vi "Role Playing Simple.vi"(0 "channel":T5, 1 "AI Parameters":T1={"GotoKick"={"Dist do cone a frente"=150.0, "attacker farback"=1500.0, "Perto"=300.0, "min dist to kick"=150.0, "kick eps"=0.0, "Time to transition"=0.05}, "Attacker"={"CC chute"=0.09, "CC passe"=0.045, "Kick Force"=100.0, "D ball-robot Kick"=200.0, "D ball-robot Pass"=0.3}, "Defender"={"D max"=1700.0, "Vel p/ robô av"=1000.0, "Kick Force"=100.0, "D atk-def"=0.0, "D farback"=0.0}, "Timeout"={"Field/v in x"=6.0, "Dist Robots"=300, "Dist up in y"=300}, "Pose Striker"={"dist"=200.0, "Numeric"=-4.0, "dist 2"=200.0}, "Dist Stop"=300.0, "Distance when ball out"=200, "D central gap "=150.0, "T pass"=0.0, "Force ++"=0.0, "range kick"=0.0, "Chute alto"=TRUE, "Marcador novo"=TRUE} {"D central gap" format="%#_13g"; "Dist Stop" format="%#_13g"; "Pose Striker"."Numeric" format="%#_13g"; "Defender"."Kick Force" format="%#_13g"; "Defender"."Vel p/ robô av" format="%#_13g"; "Attacker"."D ball-robot Kick" format="%#_13g"; "Attacker"."Kick Force" format="%#_13g"; "Attacker"."CC passe" format="%#_13g"; "Attacker"."CC chute" format="%#_13g"; "GotoKick"."kick eps" format="%#_13g"; "GotoKick"."min dist to kick" format="%#_13g"; "GotoKick"."Perto" format="%#_13g"; "GotoKick"."attacker farback" format="%#_13g"; "GotoKick"."Dist do cone a frente" format="%#_13g"}, 5 "channel":T4, 9 "test module":T2, 12 "atacando ao contrário?":bool=TRUE) -> (3 "kick \nerror":dbl, 4 "channel":T5, 6 "IA State Output":T6={"our_robots"=[], "enemy_robots"=[], "balls"=[], "geometry"={"line_width"=0, "field_length"=0, "field_width"=0, "boundary_width"=0, "referee_width"=0, "goal_width"=0, "goal_depth"=0, "goal_wall_width"=0, "center_circle_radius"=0, "defense_radius"=0, "defense_stretch"=0, "free_kick_from_defense_dist"=0, "penalty_spot_from_field_line_dist"=0, "penalty_line_from_spot_dist"=0}, "IA Judge"={"stage"="", "command"="", "our_goalie_id"=0.0, "enemy_goalie_id"=0.0, "command enum"=enum."Halt", "Time"=enum."Azul"}, "Received Timestamp"=timestamp(0 s since 1904-01-01), "Events"={"Touch"=FALSE, "Ball out"=FALSE, "id touch"=0.0, "Ball out of \nVision"=FALSE, "Ball inside \nGoalie area"=FALSE, "Robot not responding"=FALSE, "Robots responding status"=[1.0, 1.0, 1.0, 1.0, 1.0, 1.0], "Enemy Ball \nPossession"=FALSE, "Pass State"=FALSE, "id end of pass"=0.0, "Kick"=FALSE, "Id ini Possession"=0.0, "Ball Possesion"=FALSE, "Id Possesion"=0.0}}, 10 "channel to field":T5, 14 "ball":dbl(graph), 15 "Robot":dbl(graph))   [LabVIEW 2017]
uses:
  <extravilib>/ChannelInstances/Lossy Stream-t'AI Input.ctl'/)Channel.ctl
  Core/AI Input.ctl
  Core/AI Robot.ctl
  Intel/Functions Enum.ctl
  Intel/AttackerStates.ctl
  Core/AI Ball.ctl
  Core/Field Size.ctl
  Core/AI Judge.ctl
  Intel/Command Enum.ctl
  Util/Events/Events.ctl
  <extravilib>/ChannelInstances/Lossy Stream-a[.](i32)/)Channel.ctl
  Test/TestModule.ctl
  Util/Select None or Robot.ctl
  Intel/AI Parameters.ctl
  <extravilib>/ChannelInstances/Lossy Stream-a[.](i32)/Read With Abort.vi
  <extravilib>/ChannelInstances/Lossy Stream-t'AI Input.ctl'/Read With Abort.vi
  <extravilib>/ChannelInstances/Lossy Stream-t'AI Input.ctl'/Write With Abort.vi
  <extravilib>/ChannelInstances/Lossy Stream-a[.](i32)/EndpointRead.vi
  <extravilib>/ChannelInstances/Lossy Stream-t'AI Input.ctl'/EndpointRead.vi
  <extravilib>/ChannelInstances/Lossy Stream-t'AI Input.ctl'/Endpoint.vi
  <extravilib>/ChannelInstances/Lossy Stream-t'AI Input.ctl'/)Channel.vi
  <resource>/ChannelSupport/_ChannelSupport/WaitIfNeeded.vi
  <extravilib>/ChannelInstances/Lossy Stream-a[.](i32)/)Channel.vi
  <extravilib>/ChannelInstances/Lossy Stream-t'AI Input.ctl'.lvlib
  <extravilib>/ChannelInstances/Lossy Stream-a[.](i32).lvlib
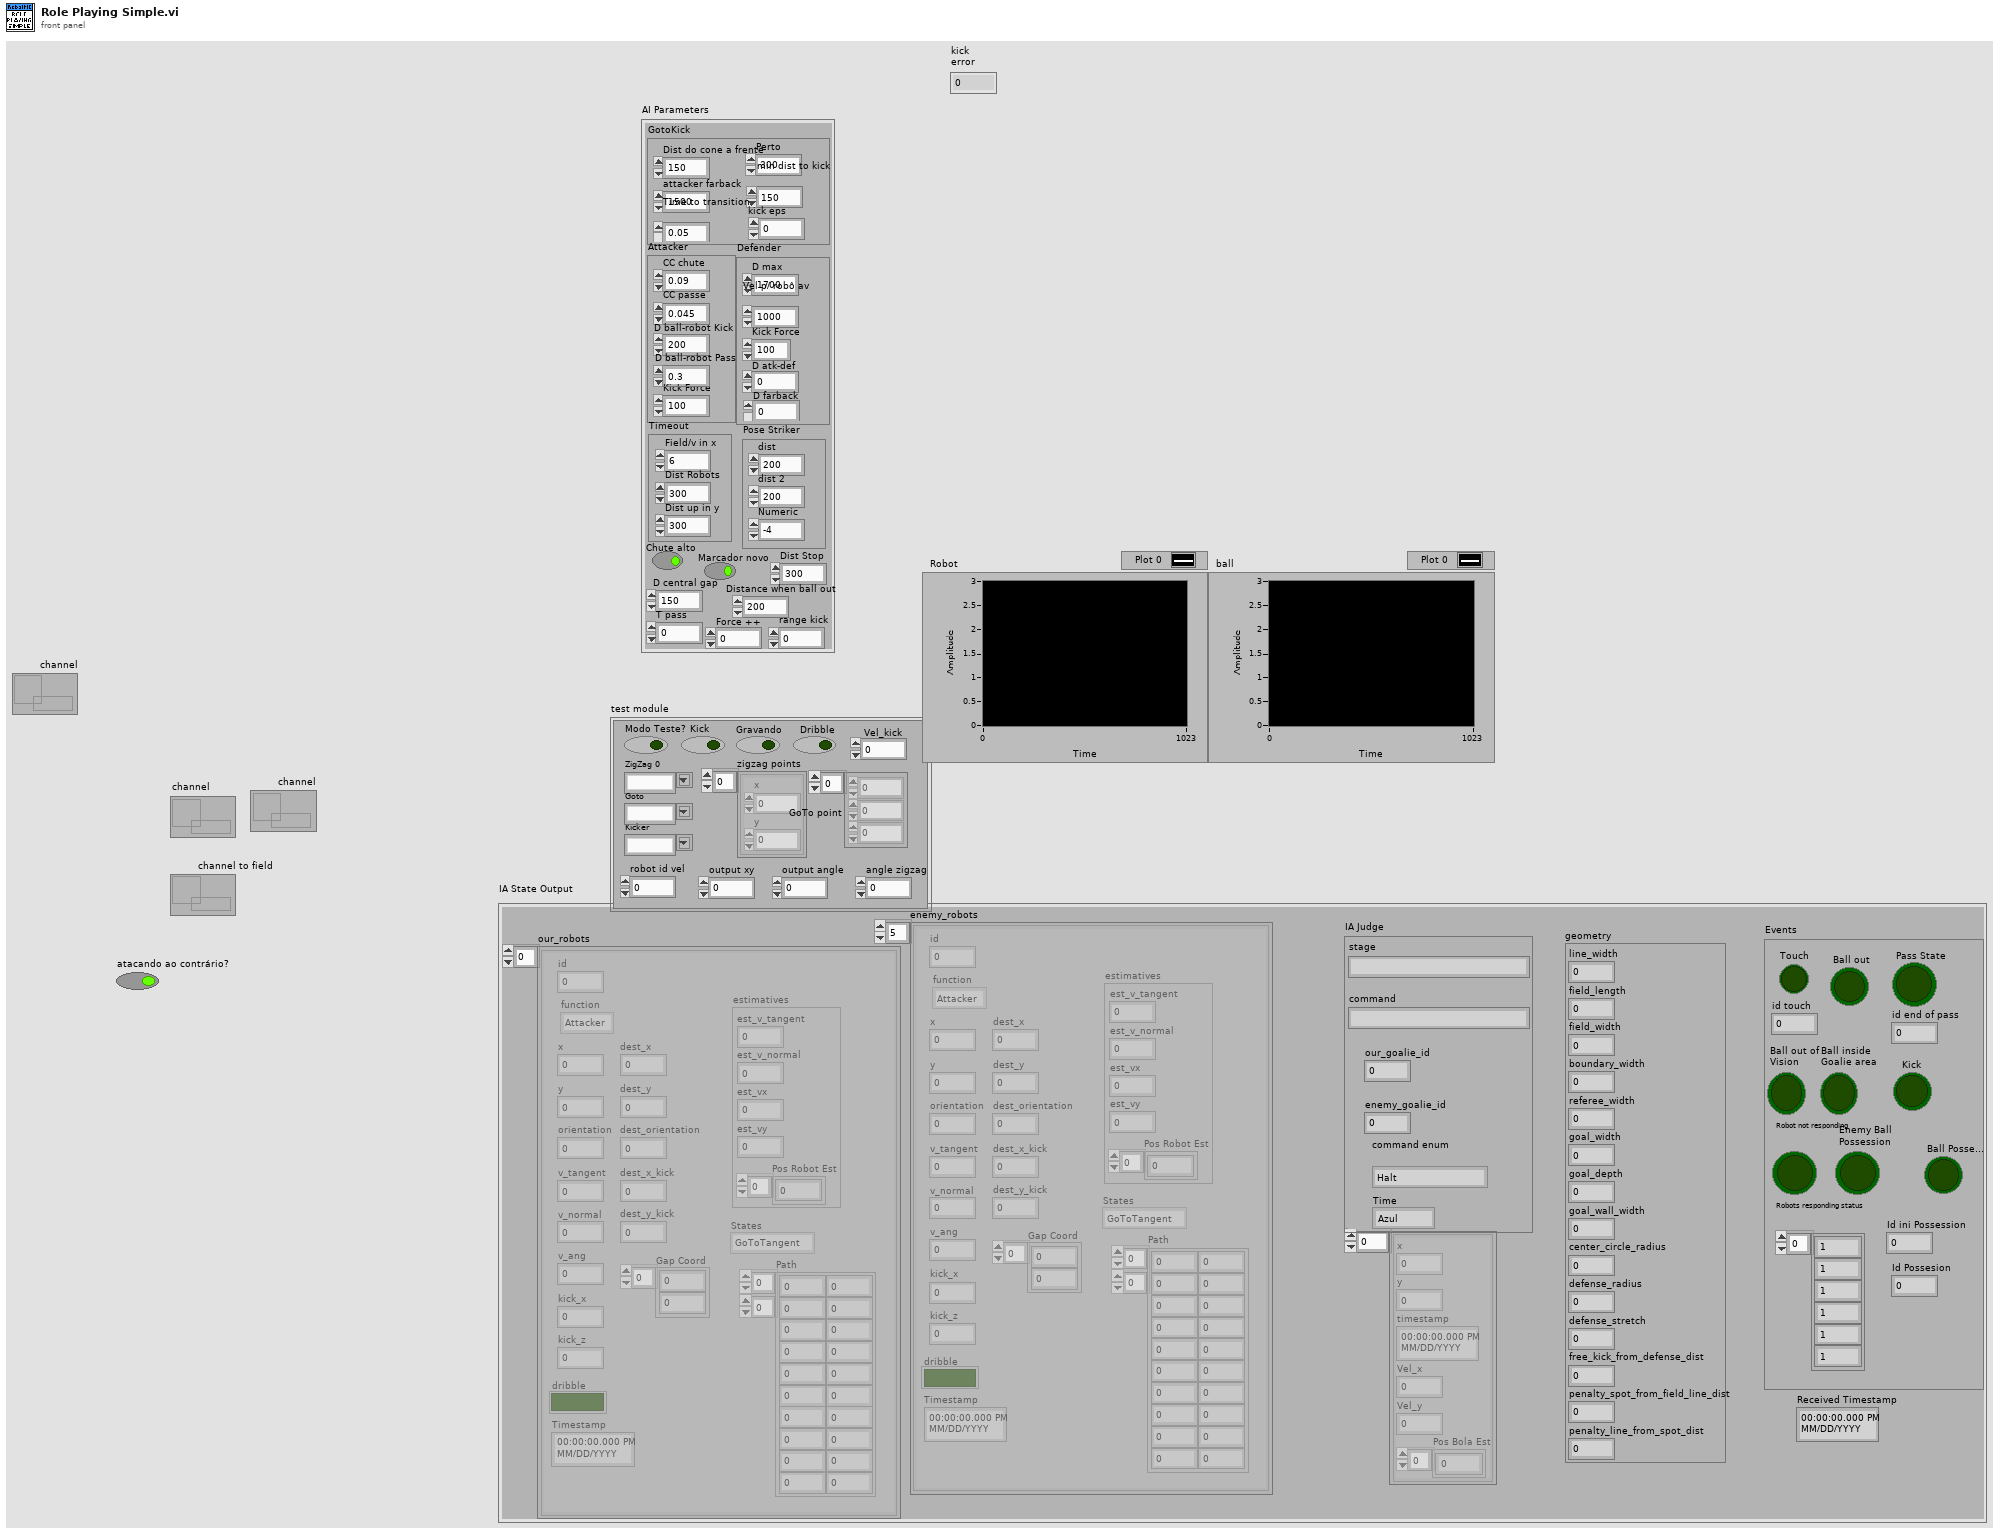
[diagram p1: front panel]
types:
  T1 = typedef "AI Parameters.ctl" = cluster{"GotoKick":cluster{"Dist do cone a frente":dbl, "attacker farback":dbl, "Perto":dbl, "min dist to kick":dbl, "kick eps":dbl, "Time to transition":dbl}, "Attacker":cluster{"CC chute":dbl, "CC passe":dbl, "Kick Force":dbl, "D ball-robot Kick":dbl, "D ball-robot Pass":dbl}, "Defender":cluster{"D max":dbl, "Vel p/ robô av":dbl, "Kick Force":dbl, "D atk-def":dbl, "D farback":dbl}, "Timeout":cluster{"Field/v in x":dbl, "Dist Robots":u32, "Dist up in y":u32}, "Pose Striker":cluster{"dist":dbl, "Numeric":dbl, "dist 2":dbl}, "Dist Stop":dbl, "Distance when ball out":i32, "D central gap ":dbl, "T pass":dbl, "Force ++":dbl, "range kick":dbl, "Chute alto":bool, "Marcador novo":bool}
  T2 = typedef "TestModule.ctl" = cluster{"Goto":T3, "ZigZag 0":T3, "Kicker":T3, "Vel_kick":dbl, "Kick":bool, "Modo Teste?":bool, "GoTo point":dbl[], "zigzag points":cluster{"x":dbl, "y":dbl}[], "robot id vel":u32, "Dribble":bool, "Gravando":bool, "output xy":dbl, "output angle":dbl, "angle zigzag":dbl}
  T3 = typedef "Select None or Robot.ctl" = string
  T4 = typedef "Lossy Stream-a[.](i32).lvlib/)Channel.ctl" = refnum<queue>
  T5 = typedef "Lossy Stream-t'AI Input.ctl'.lvlib/)Channel.ctl" = refnum<queue>
  T6 = typedef "AI Input.ctl" = cluster{"our_robots":T7[], "enemy_robots":T7[], "balls":T10[], "geometry":T11, "IA Judge":T12, "Received Timestamp":timestamp, "Events":T14}
  T7 = typedef "AI Robot.ctl" = cluster{"id":u32, "function":T8, "x":dbl, "y":dbl, "orientation":dbl, "v_tangent":dbl, "v_normal":dbl, "v_ang":dbl, "kick_x":dbl, "kick_z":dbl, "dribble":bool, "Timestamp":timestamp, "dest_x":dbl, "dest_y":dbl, "dest_orientation":dbl, "estimatives":cluster{"est_v_tangent":dbl, "est_v_normal":dbl, "est_vx":dbl, "est_vy":dbl, "Pos Robot Est":dbl[]}, "dest_x_kick":dbl, "dest_y_kick":dbl, "Gap Coord":dbl[], "States":T9, "Path ":dbl[][]}
  T8 = typedef "Functions Enum.ctl" = enum16{"Attacker", "Goalie", "Defender", "Striker", "Goto 0", "Dummy", "Kicker", "ZigZag"}
  T9 = typedef "AttackerStates.ctl" = enum16{"Pass", "GoToTangent", "BallGetting", "GoToKick", ""}
  T10 = typedef "AI Ball.ctl" = cluster{"x":dbl, "y":dbl, "timestamp":timestamp, "Vel_x":dbl, "Vel_y":dbl, "Pos Bola Est":dbl[]}
  T11 = typedef "Field Size.ctl" = cluster{"line_width":u32, "field_length":u32, "field_width":u32, "boundary_width":u32, "referee_width":u32, "goal_width":u32, "goal_depth":u32, "goal_wall_width":u32, "center_circle_radius":u32, "defense_radius":u32, "defense_stretch":u32, "free_kick_from_defense_dist":u32, "penalty_spot_from_field_line_dist":u32, "penalty_line_from_spot_dist":u32}
  T12 = typedef "AI Judge.ctl" = cluster{"stage":string, "command":string, "our_goalie_id":dbl, "enemy_goalie_id":dbl, "command enum":T13, "Time":enum16{"Azul", "Amarelo"}}
  T13 = typedef "Command Enum.ctl" = enum16{"Halt", "Stop", "Force Start", "PKA Normal Start", "Prepare Kickoff Ally", "PKE Normal Start", "Prepare Kickoff Enemy", "Prepare Penalty Ally", "PPA Normal Start", "Prepare Penalty Enemy", "PPE Normal Start", "Direct Free Enemy", "Direct Free Ally", "Indirect Free Enemy", "Indirect Free Ally", "Timeout Enemy", "Timeout Ally", "Goal Enemy", "Goal Ally", "Ball Placement Enemy", "Ball Placement Ally", "Normal Half Time", "Extra Time Break", "Extra Half Time", "None", "Post Game"}
  T14 = typedef "Events.ctl" = cluster{"Touch":bool, "Ball out":bool, "id touch":dbl, "Ball out of \nVision":bool, "Ball inside \nGoalie area":bool, "Robot not responding":bool, "Robots responding status":dbl[], "Enemy Ball \nPossession":bool, "Pass State":bool, "id end of pass":dbl, "Kick":bool, "Id ini Possession":dbl, "Ball Possesion":bool, "Id Possesion":dbl}
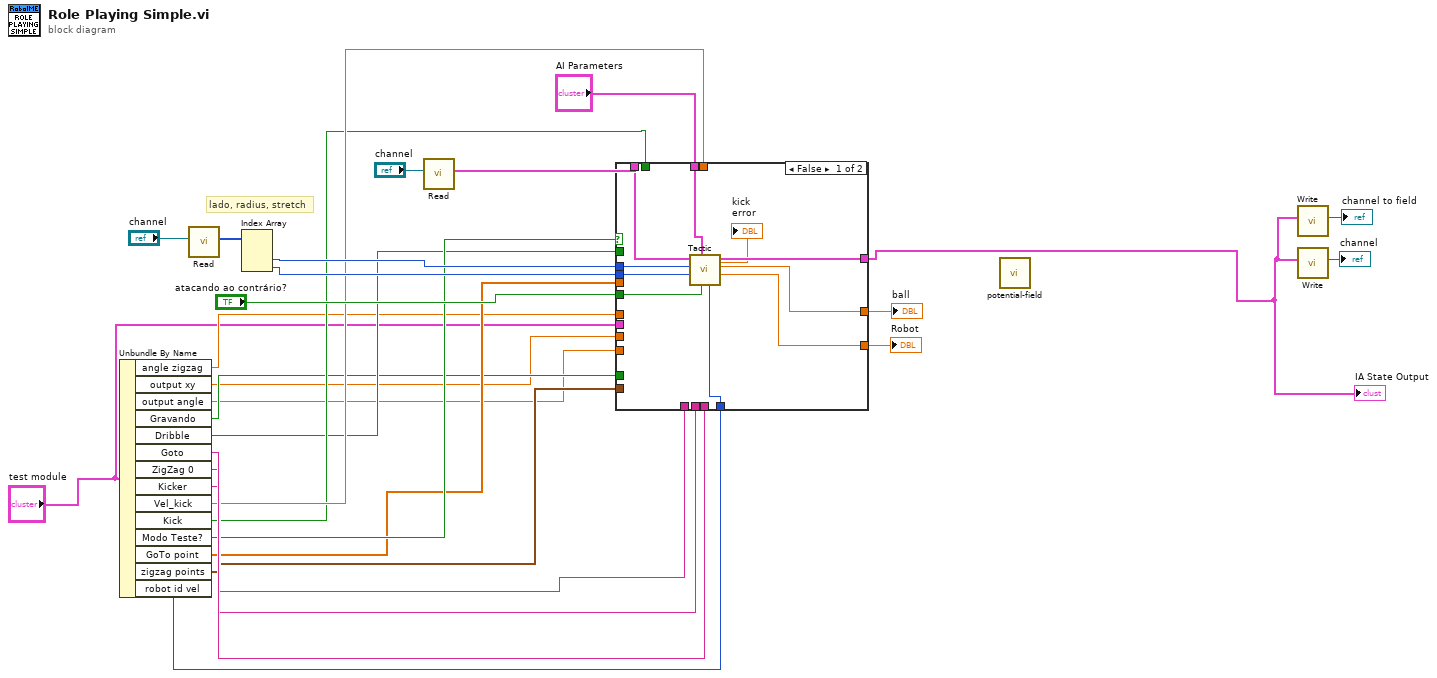
[diagram p0: block diagram]
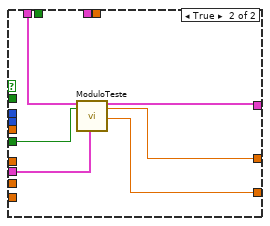
[diagram p2: hidden frame]
diagram:
  # "lado, radius, stretch"
  n1 = Unbundle By Name("test module") -> ("angle zigzag"=w3:dbl, "output xy"=w5:dbl, "output angle"=w4:dbl, "Gravando"=w9:bool, "Dribble"=w10:bool, "Goto"=w19:T3, "ZigZag 0"=w18:T3, "Kicker"=w17:T3, "Vel_kick"=w16:dbl, "Kick"=w15:bool, "Modo Teste?"=w14:bool, "GoTo point"=w13:dbl[], "zigzag points"=w12:cluster{"x":dbl, "y":dbl}[], "robot id vel"=w11:u32)
  n2 = call <extravilib>:"Read.vi"("channel"="channel") -> ("element"=w22:i32[])  [unwired: 5 in, 5 out]
  n3 = Index Array(array=w22) -> (element #2=w20:i32, element #3=w21:i32)  [unwired: 3 in, 1 out]
  n4 = call <extravilib>:"Read.vi"("channel"="channel") -> ("element"=w27:T6)  [unwired: 5 in, 5 out]
  n5 = case shown="False" w14 {
    tunnel: w27 -> [w38 w43]
    tunnel: [w37 w44] -> w2
    tunnel: w12 -> [_ _]
    tunnel: w13 -> [_ _]
    tunnel: "atacando ao contrário?" -> [w36 w42]
    tunnel: w20 -> [w35 _]
    tunnel: w21 -> [w34 _]
    tunnel: w18 -> [_ _]
    tunnel: w19 -> [_ _]
    tunnel: w16 -> [_ _]
    tunnel: w15 -> [_ _]
    tunnel: w17 -> [_ _]
    tunnel: w11 -> [w30 _]
    tunnel: [w33 w41] -> w7
    tunnel: w10 -> [_ _]
    tunnel: w9 -> [_ _]
    tunnel: [w32 w40] -> w8
    tunnel: "AI Parameters" -> [w31 _]
    tunnel: w5 -> [_ _]
    tunnel: w4 -> [_ _]
    tunnel: w3 -> [_ _]
    tunnel: "test module" -> [_ w39]
    frame False {
      n6 = call "Tactic.vi"("robot id vel"=w30, "atacando ao contrário?"=w36, "AI Parameters"=w31, "Defense stretch"=w34, "Defense radius"=w35, "IA State Input"=w38) -> ("Robot"=w32:dbl, "ball"=w33:dbl, "IA State Output"=w37:T6, "kick \nerror"=→"kick \nerror":dbl)  [unwired: 2 in]
    }
    frame True {
      n7 = call "ModuloTeste.vi"("IA State Input"=w43, "atacando ao contrário?"=w42, "test module"=w39) -> ("IA State Output"=w44:T6, "ball"=w41:dbl, "Robot"=w40:dbl)  [unwired: 14 in]
    }
  }
  "IA State Output" <- w2
  "ball" <- w7
  "Robot" <- w8
  n8 = call "potential-field.vi"() -> ()  [unwired: 11 in, 1 out]
  n9 = call <extravilib>:"Write.vi"("element"=w2) -> ("channel"=→"channel to field":T5)  [unwired: 8 in, 2 out]
  n10 = call <extravilib>:"Write.vi"("element"=w2) -> ("channel"=→"channel":T5)  [unwired: 8 in, 2 out]
